vi "Main.vi"() -> ()   [LabVIEW 2017]
doc: "This sample project is built upon the standard state machine template and shows how you could create an application that acquires, analyzes, and presents data. It includes functionality for presenting configuration dialogs, preserving settings between executions, loading and saving data, as well as exporting graph images and text files.\n\nIt is most appropriate for data that is acquired instantly as it does not allow for screen updates mid acquisition nor does it allow for continuous streaming to disk."
uses:
  controls/State.ctl
  controls/Data.ctl
  controls/UI References.ctl
  controls/Graph Data.ctl
  <vilib>/Utility/miscctls.llb/LVAnnotationListTypeDef.ctl
  <vilib>/Utility/miscctls.llb/LVCursorListTypeDef.ctl
  controls/User Specified Data.ctl
  controls/HW Configuration.ctl
  original/controls/Simulated Signal Type.ctl
  controls/Analysis Configuration.ctl
  controls/New Data Behavior.ctl
  <extravilib>/ChannelInstances/Event Messenger-a[.](str)/Instantiate.vi
  <extravilib>/ChannelInstances/Event Messenger-a[.](str)/))Channel.vi
  <extravilib>/ChannelInstances/Event Messenger-str/Instantiate.vi
  <extravilib>/ChannelInstances/Event Messenger-str/))Channel.vi
  subVIs/Settings Dialog.vi
  <extravilib>/ChannelInstances/Event Messenger-str.lvlib
  <extravilib>/ChannelInstances/Event Messenger-a[.](str).lvlib
panel:
  in  "Settings":bool
  in  "Snapshot":bool
  in  "Analyze":bool
  in  "Clear":bool
  in  "Exit":bool
  in  "Acquire":bool
  in  "Export":bool
  in  "Save Data":bool
  in  "Load Data":bool
  out "Graph":waveform(dbl)[](graph)
  out "Status Bar":string
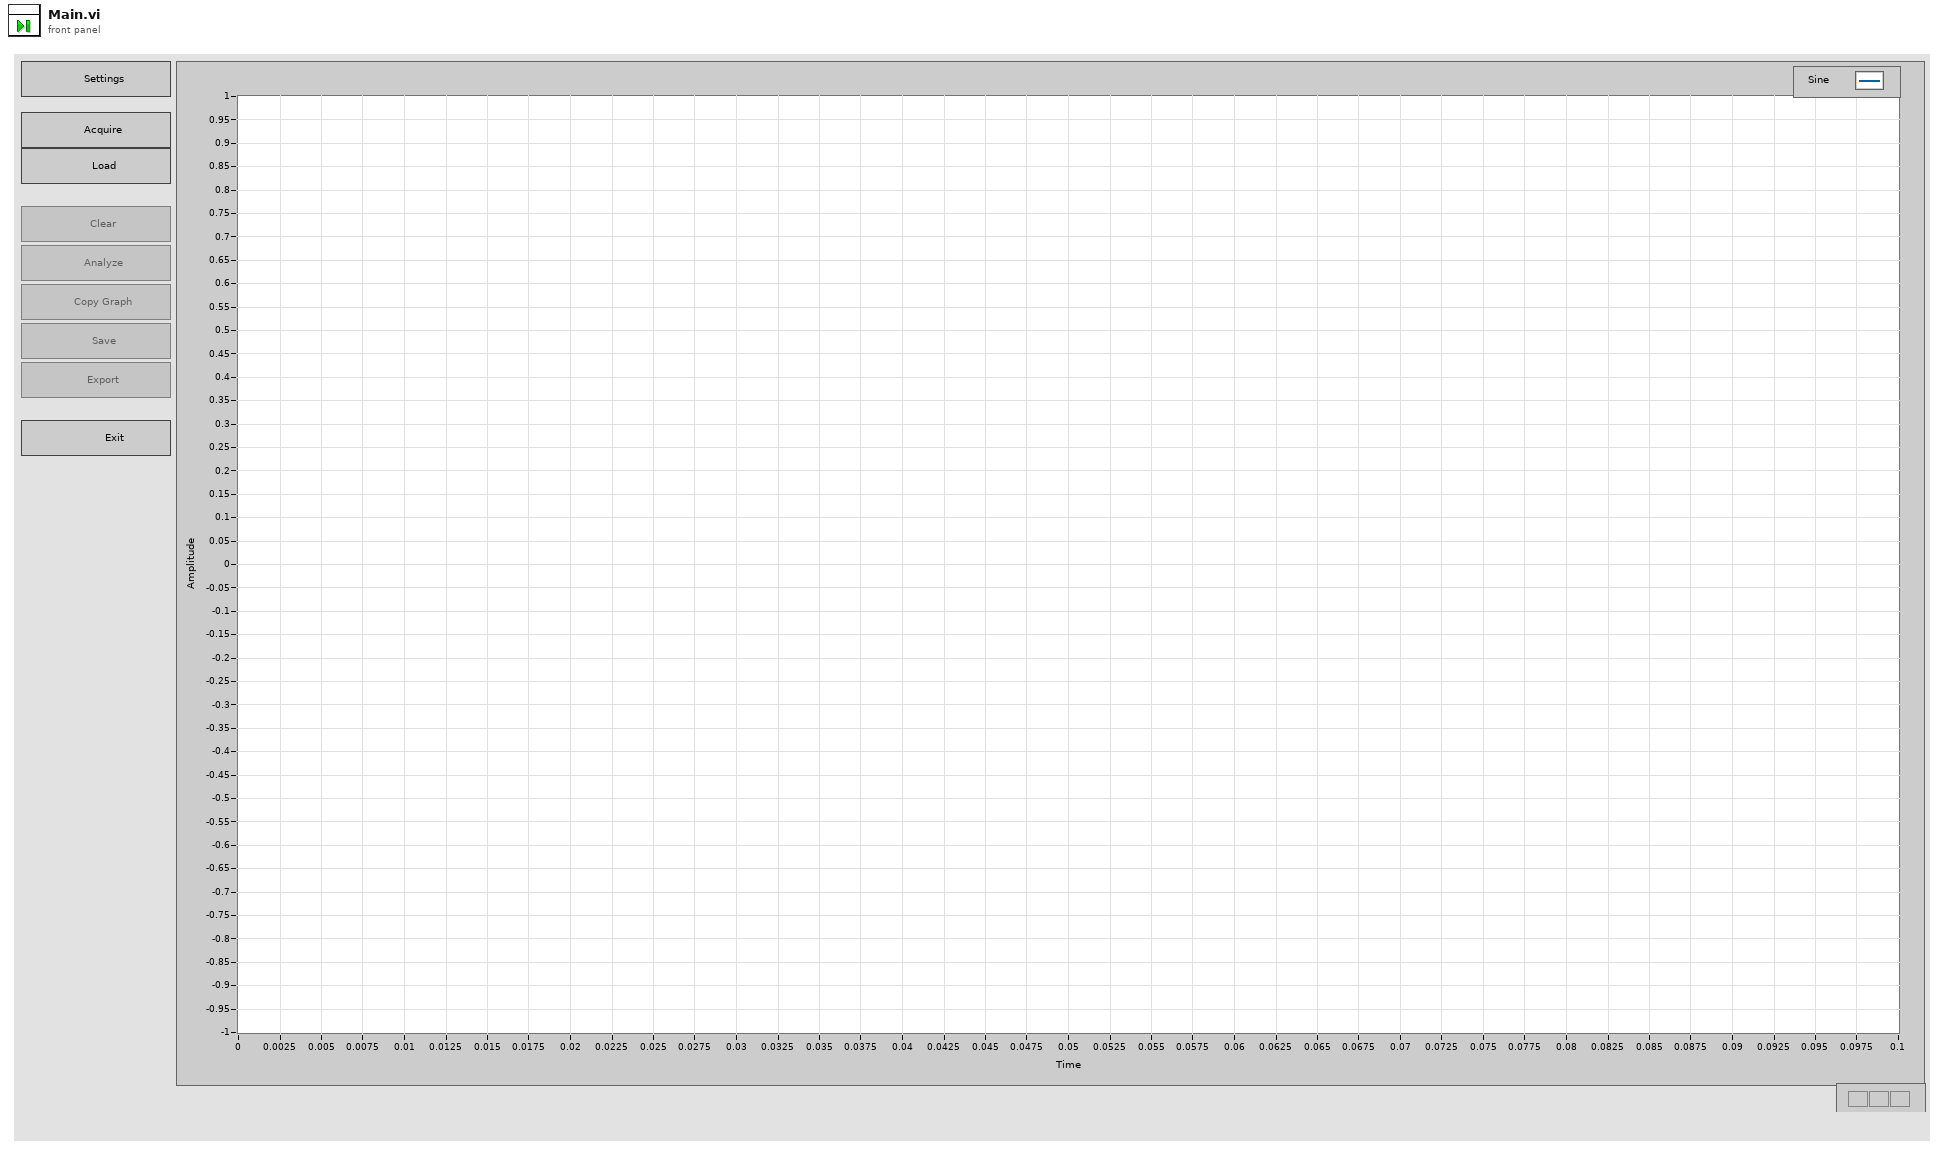
[diagram p1: front panel]
types:
  T1 = typedef "Data.ctl" = cluster{"UI References":T2, "Graph Data":T3, "User Specified":T6}
  T2 = typedef "UI References.ctl" = cluster{"Exit Ref":refnum<vi>, "Save Ref":refnum<vi>, "Open Ref":refnum<vi>, "Export Ref":refnum<vi>, "Acquire Ref":refnum<vi>, "Configure Ref":refnum<vi>, "Graph Ref":refnum<vi>, "Clear Ref":refnum<vi>, "Analyze Ref":refnum<vi>, "Status Ref":refnum<vi>, "Snapshot Ref":refnum<vi>}
  T3 = typedef "Graph Data.ctl" = cluster{"Data":waveform(dbl)[], "Annotation List":T4, "Cursor List":T5, "Analysis Data":waveform(dbl)[]}
  T4 = typedef "LVAnnotationListTypeDef.ctl" = cluster{"Name":string, "Color":u32, "Style":u8, "Point Style":u8, "Name Visible":bool, "Allow Drag":bool, "Annotation Mode":u32, "Plot":i32, "Index":i32, "Position":cluster{"X":dbl, "Y":dbl}, "X Scale":u32, "Y Scale":u32, "Show Arrow":bool, "Lock Name":bool, "Plot Area":i32, "Label Offset":cluster{"X":dbl, "Y":dbl}}[]
  T5 = typedef "LVCursorListTypeDef.ctl" = cluster{"Name":string, "Color":u32, "Style":u8, "Point Style":u8, "Name Visible":bool, "Allow Drag":bool, "Cursor Mode":u32, "Plot":i32, "Index":i32, "Position":cluster{"X":dbl, "Y":dbl}, "X Scale":u32, "Y Scale":u32, "Watch Plots":i32[], "Watch All Plots":bool, "Plot Area":i32, "Label Offset":cluster{"X":dbl, "Y":dbl}}[]
  T6 = typedef "User Specified Data.ctl" = cluster{"Hardware Configuration":T7, "Analysis Configuration":T9, "New Data Behavior":T10, "Signal Configuration":cluster{"I/O Limit":dbl, "Sample Rate":dbl, "Chirp Duration (s)":dbl, "Upper Frequency":dbl, "Lower Frequency":dbl, "Chirp Amplitude":dbl, "Windowing":enum16{"None", "Exponential", "Flat top", "Hamming", "Hanning", "Kaiser-Bessel", "Rectangular"}}}
  T7 = typedef "HW Configuration.ctl" = cluster{"Signal Channel":tag, "Response Channel":tag, "Trigger Channel":tag, "HW Refnum <Replace Me>":string, "Signal Type <Replace Me>":T8}
  T8 = typedef "Simulated Signal Type.ctl" = enum16{"Sine Wave", "Square Wave"}
  T9 = typedef "Analysis Configuration.ctl" = cluster{"Statistics":bool}
  T10 = typedef "New Data Behavior.ctl" = enum16{"Replace", "Overlay", "Append"}
  T11 = typedef "State.ctl" = enum16{"Initialize", "Wait for Event", "Update UI", "Configure", "Acquire", "Load Data", "Save Data", "Clear Data", "Export Data", "Analyze", "Copy Graph", "Exit"}
  T12 = enum16{"Standard", "Buffered", "CRLF", "Immediate"}
  T13 = typedef "Event Messenger-str.lvlib/))Channel.ctl" = refnum<queue>
  T14 = typedef "Event Messenger-a[.](str).lvlib/))Channel.ctl" = refnum<queue>
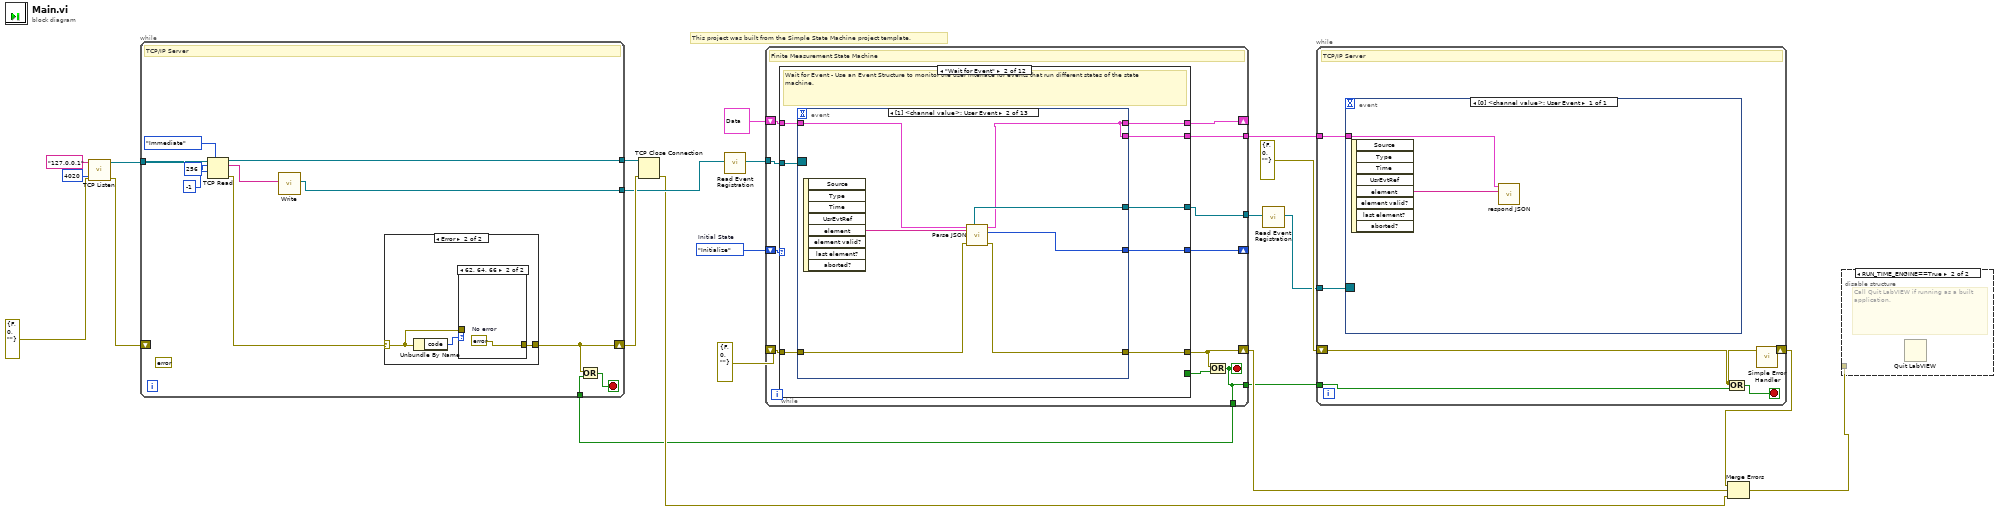
[diagram p0: block diagram]
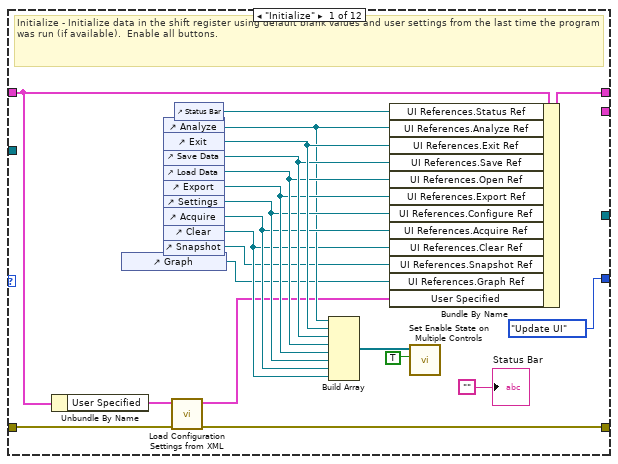
[diagram p5: hidden frame]
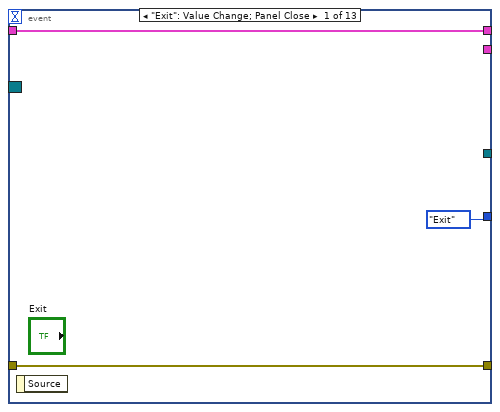
[diagram p6: hidden frame]
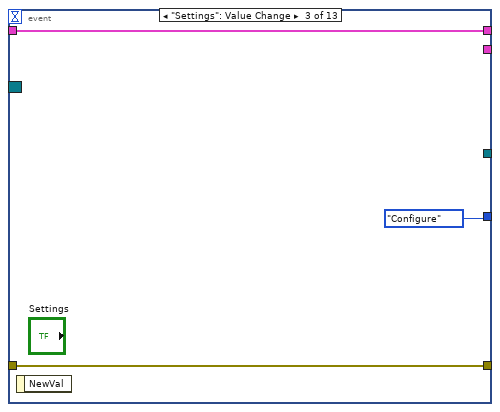
[diagram p7: hidden frame]
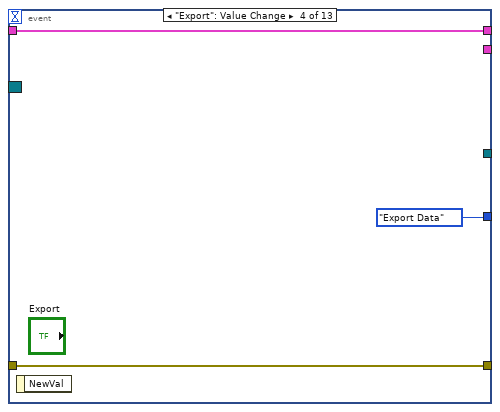
[diagram p8: hidden frame]
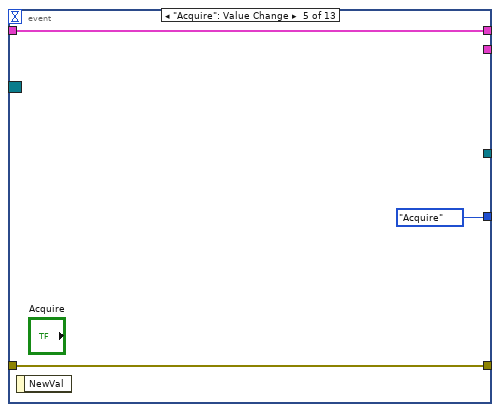
[diagram p9: hidden frame]
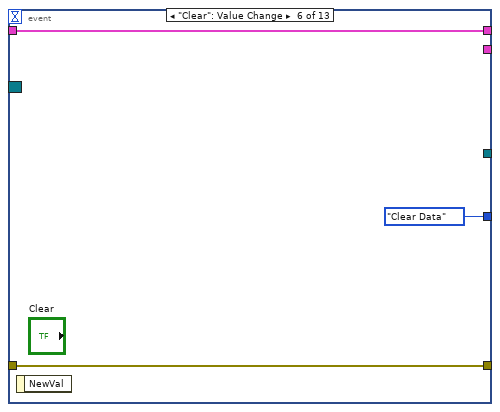
[diagram p10: hidden frame]
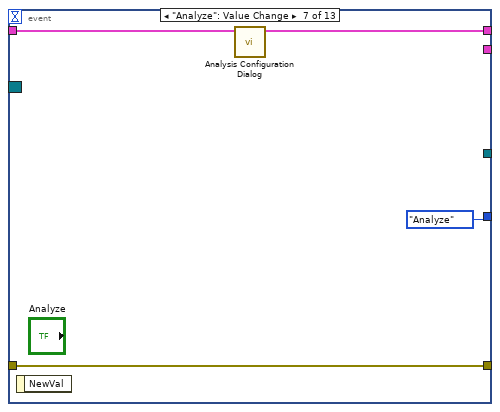
[diagram p11: hidden frame]
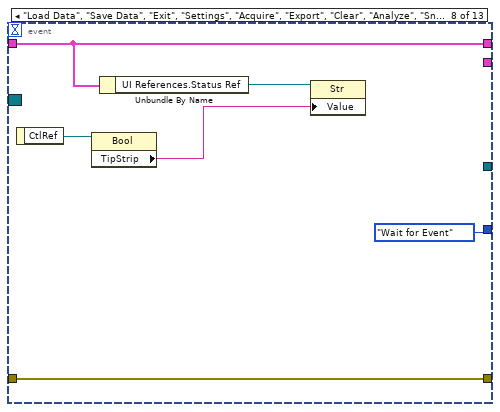
[diagram p12: hidden frame]
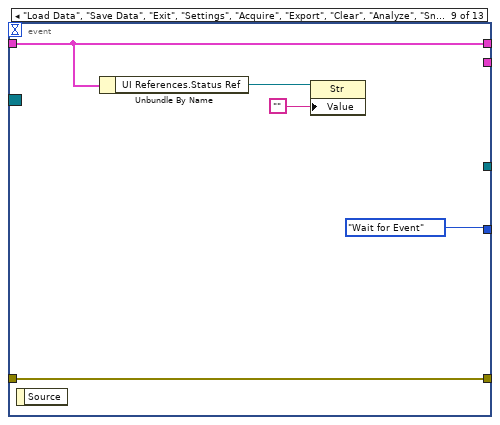
[diagram p13: hidden frame]
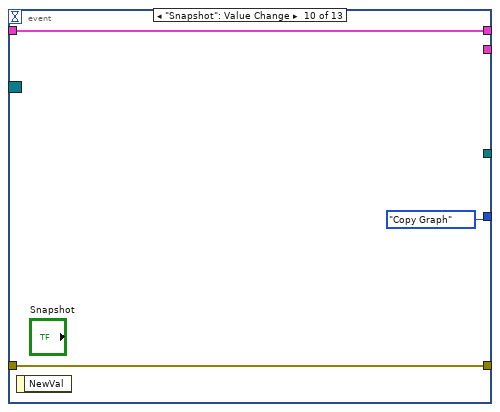
[diagram p14: hidden frame]
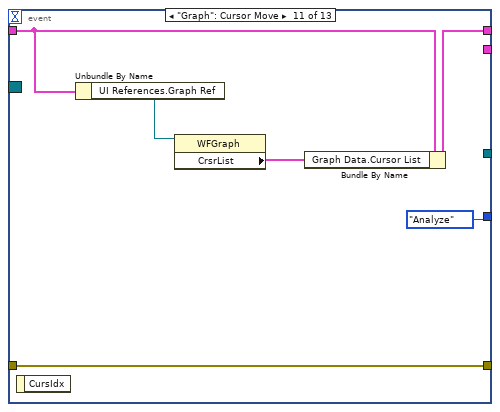
[diagram p15: hidden frame]
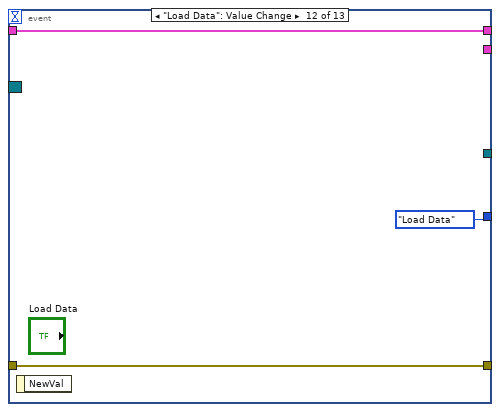
[diagram p16: hidden frame]
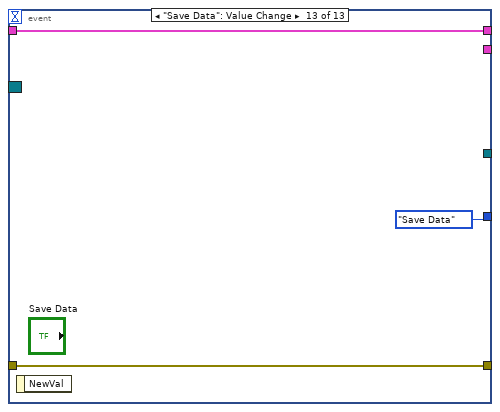
[diagram p17: hidden frame]
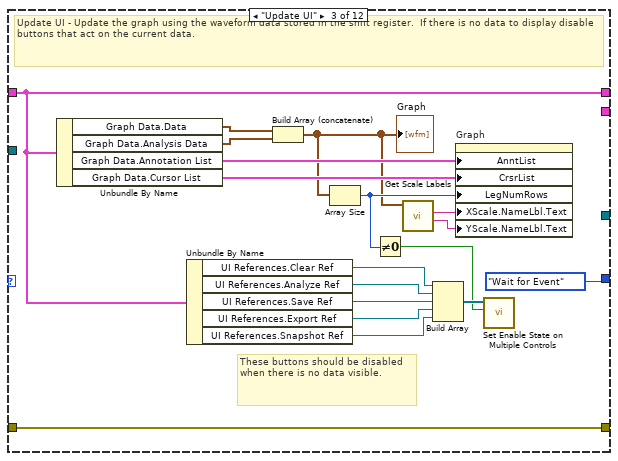
[diagram p18: hidden frame]
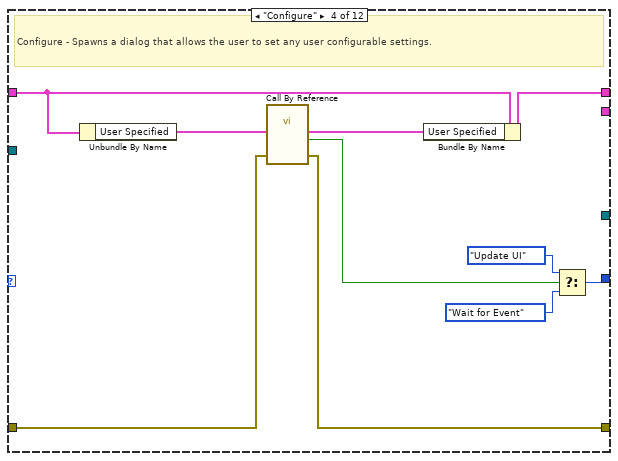
[diagram p19: hidden frame]
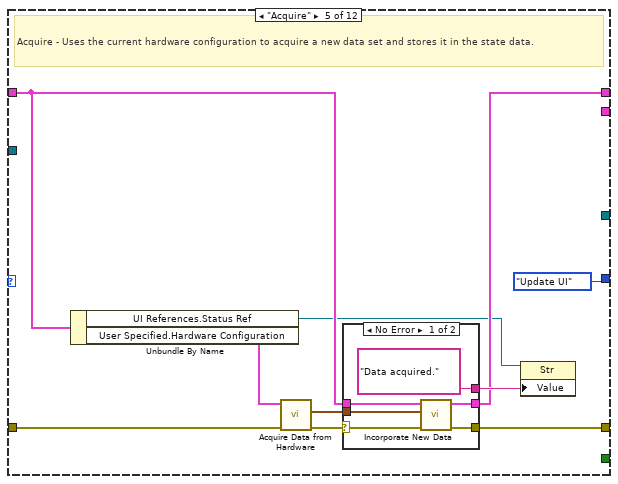
[diagram p20: hidden frame]
diagram:
  (unwired) errorcluster {"status"=FALSE, "code"=0, "source"=""} ("error constant")
  w22 = State."Initialize"  # Initial State
  # "This project was built from the Simple State Machine project template."
  n1 = call <vilib>:"TCP Listen.vi"("error in (no error)"=errorcluster {"status"=FALSE, "code"=0, "source"=""} ("error constant"), "port"=u16 4020 ("remote port or service name"), "service name"="127.0.0.1" ("address")) -> ("error out"=w11:errorcluster, "connection ID"=w18:refnum<k5>)  [unwired: 4 in, 3 out]
  n2 = call <vilib>:"Simple Error Handler.vi"() -> ()  [unwired: 5 in, 5 out]
  n3 = while {
    tunnel: w18 -> [w32]
    tunnel: [w28] -> w17
    tunnel: [w26] -> w15
    shift-right: [w24] -> w16
    shift-left: w11 -> [_]
    tunnel: w1 -> [w23]
    stop <- w33 stop-if-true
    # "TCP/IP Server"
    n4 = TCP Read(connection ID=w32, bytes to read=256, 7:T12."Immediate" ("mode (standard)"), 9:-1 ("timeout ms (25000)")) -> (connection ID out=w28:refnum<k5>, data out=w27:string, error out=w25:errorcluster)  [unwired: 1 in]
    n5 = call <extravilib>:"Write.vi"("element"=w27) -> ("channel"=w26:T13)  [unwired: 9 in, 1 out]
    n6 = case shown="Error" w25 {
      selector: w25 -> [w34 w35]
      tunnel: [w34 w36] -> w24
      frame No Error {
      }
      frame Error {
        n7 = Unbundle By Name(w35) -> ("code"=w37:i32)
        n8 = case shown="62, 64, 66" w37 {
          tunnel: [w38 w39] -> w36
          tunnel: w35 -> [w38 _]
          frame 0, Default {
          }
          frame 62, 64, 66 {
            w39 = errorcluster {"status"=FALSE, "code"=0, "source"=""}  # No error
          }
        }
      }
    }
    n9 = Or(x=w24, y=w23) -> (x .or. y?=w33:bool)
  }
  n10 = TCP Close Connection(connection ID=w17, error in (no error)=w16) -> (error out=w8:errorcluster)  [unwired: 2 out]
  n11 = call <extravilib>:"Read Event Registration.vi"("channel"=w15) -> ("event registration refnum"=w14:refnum<event-registration>)  [unwired: 10 in]
  n12 = while {
    shift-right: [w42] -> _
    shift-left: w22 -> [w50]
    shift-right: [w48] -> _
    shift-left: T1 {"UI References"={"Exit Ref"=refnum, "Save Ref"=refnum, "Open Ref"=refnum, "Export Ref"=refnum, "Acquire Ref"=refnum, "Configure Ref"=refnum, "Graph Ref"=refnum, "Clear Ref"=refnum, "Analyze Ref"=refnum, "Status Ref"=refnum, "Snapshot Ref"=refnum}, "Graph Data"={"Data"=[], "Annotation List"=[], "Cursor List"=[], "Analysis Data"=[]}, "User Specified"={"Hardware Configuration"={"Signal Channel"="", "Response Channel"="", "Trigger Channel"="", "HW Refnum <Replace Me>"="", "Signal Type <Replace Me>"=enum."Sine Wave"}, "Analysis Configuration"={"Statistics"=TRUE}, "New Data Behavior"=enum."Replace", "Signal Configuration"={"I/O Limit"=10.0, "Sample Rate"=1000000.0, "Chirp Duration (s)"=0.01, "Upper Frequency"=0.0, "Lower Frequency"=0.0, "Chirp Amplitude"=0.1, "Windowing"=enum."None"}}} ("Data") -> [w49]
    shift-right: [w45] -> w7
    shift-left: errorcluster {"status"=FALSE, "code"=0, "source"=""} ("error constant") -> [w47]
    tunnel: w14 -> [w44]
    tunnel: [w43] -> w5
    tunnel: [w41] -> w3
    tunnel: [w40] -> w2
    tunnel: [w40] -> w1
    stop <- w40 stop-if-true
    # "Finite Measurement State Machine"
    n13 = case shown="\"Wait for Event\"" w50 {
      tunnel: [_ w79 _ _ _ _ _ _ _ _ _ _] -> w43
      tunnel: [_ _ _ _ _ _ _ _ _ _ _ w241] -> w46
      tunnel: w49 -> [w63 w78 w147 w159 w166 w187 w201 w213 w224 w227 w233 w239]
      tunnel: [w71 w77 w147 w158 w165 w182 w201 w213 w223 w227 w233 w239] -> w48
      tunnel: w47 -> [w61 w76 w149 w157 w168 w186 w203 w216 w225 w228 w232 w236]
      tunnel: [w60 w75 w149 w156 w161 w185 w199 w210 w225 w228 w231 w235] -> w45
      tunnel: w44 -> [_ w74 _ _ _ _ _ _ _ _ _ _]
      tunnel: [State."Update UI" ("Next State") w73 State."Wait for Event" ("(Value Not Used)") w150 State."Update UI" ("Next State") State."Update UI" ("(Value Not Used)") State."Wait for Event" ("(Value Not Used)") State."Wait for Event" ("(Value Not Used)") State."Update UI" ("(Value Not Used)") State."Update UI" ("(Value Not Used)") State."Wait for Event" ("(Value Not Used)") w234] -> w42
      tunnel: [_ w72 _ _ _ _ _ _ _ _ _ _] -> w41
      frame "Initialize" {
        # "Initialize - Initialize data in the shift register using default blank values and user settings from the last time the program was run (if available).  Enable all buttons."
        n14 = Unbundle By Name(w63) -> ("User Specified"=w62:T6)
        n15 = control-ref of="Graph"() -> (w52:refnum<vi>)
        n16 = control-ref of="Analyze"() -> (w59:refnum<vi>)
        n17 = control-ref of="Exit"() -> (w70:refnum<vi>)
        n18 = control-ref of="Save Data"() -> (w69:refnum<vi>)
        n19 = control-ref of="Load Data"() -> (w68:refnum<vi>)
        n20 = control-ref of="Export"() -> (w67:refnum<vi>)
        n21 = control-ref of="Settings"() -> (w66:refnum<vi>)
        n22 = control-ref of="Acquire"() -> (w65:refnum<vi>)
        n23 = control-ref of="Clear"() -> (w57:refnum<vi>)
        n24 = control-ref of="Snapshot"() -> (w53:refnum<vi>)
        n25 = call "Load Configuration Settings from XML.vi"("error in (no error)"=w61, "User Configuration in"=w62) -> ("error out"=w60:errorcluster, "User Configuration out"=w55:T6)  [unwired: 8 in]
        n26 = control-ref of="Status Bar"() -> (w58:refnum<vi>)
        n27 = Build Array(w59, w70, w69, w68, w67, w66, w65, w57) -> (w64:refnum<vi>[])
        n28 = Bundle By Name(cluster=w63, "UI References.Status Ref"=w58, "UI References.Analyze Ref"=w59, "UI References.Exit Ref"=w70, "UI References.Save Ref"=w69, "UI References.Open Ref"=w68, "UI References.Export Ref"=w67, "UI References.Configure Ref"=w66, "UI References.Acquire Ref"=w65, "UI References.Clear Ref"=w57, "UI References.Snapshot Ref"=w53, "UI References.Graph Ref"=w52, "User Specified"=w55) -> (w71:T1)
        n29 = call "Set Enable State on Multiple Controls.vi"("Enable?"=TRUE, "Controls"=w64) -> ()  [unwired: 10 in]
        "Status Bar" <- "" ("Status Bar")
      }
      frame "Wait for Event" {
        # "Wait for Event - Use an Event Structure to monitor the user interface for events that run different states of the state machine."
        n30 = event shown="[1] <channel value>: User Event" {
          selector: w74 -> [_ _ _ _ _ _ _ _ _ _ _ _ _]
          dyn-events: _ -> [_ _ _ _ _ _ _ _ _ _ _ _ _]
          timeout: _ -> [_ _ _ _ _ _ _ _ _ _ _ _ _]
          tunnel: [_ w85 _ _ _ _ _ _ _ _ _ _ _] -> w79
          tunnel: w78 -> [w82 w88 w92 w95 w98 w101 w104 w109 w115 w119 w121 w128 w131]
          tunnel: [w82 w83 w92 w95 w98 w101 w103 w109 w115 w119 w124 w128 w131] -> w77
          tunnel: w76 -> [w81 w87 w91 w94 w97 w100 w105 w111 w116 w118 w125 w127 w130]
          tunnel: [w81 w86 w91 w94 w97 w100 w105 w111 w116 w118 w125 w127 w130] -> w75
          tunnel: [State."Exit" ("Next State") w84 State."Configure" ("Next State") State."Export Data" ("Next State") State."Acquire" ("Next State") State."Clear Data" ("Next State") State."Analyze" ("Next State") State."Wait for Event" ("Next State") State."Wait for Event" ("Next State") State."Copy Graph" ("Next State") State."Analyze" ("Next State") State."Load Data" ("Next State") State."Save Data" ("Next State")] -> w73
          tunnel: [_ w83 _ _ _ _ _ _ _ _ _ _ _] -> w72
          event "Exit": Value Change; Panel Close {
            n31 = event-data() -> ()  [unwired: 1 in, 1 out]
          }
          event User Event {
            n32 = event-data() -> ("element"=w89:string)  [unwired: 1 in, 7 out]
            n33 = call "Parse JSON.vi"("error in (no error)"=w87, "element"=w89, "Data In"=w88) -> ("error in (no error) 2"=w86:errorcluster, "States"=w84:T11, "Data Out"=w83:T1, "Message Channel"=w85:T14)  [unwired: 3 in]
          }
          event "Settings": Value Change {
            n34 = event-data() -> ()  [unwired: 1 in, 1 out]
          }
          event "Export": Value Change {
            n35 = event-data() -> ()  [unwired: 1 in, 1 out]
          }
          event "Acquire": Value Change {
            n36 = event-data() -> ()  [unwired: 1 in, 1 out]
          }
          event "Clear": Value Change {
            n37 = event-data() -> ()  [unwired: 1 in, 1 out]
          }
          event "Analyze": Value Change {
            n38 = event-data() -> ()  [unwired: 1 in, 1 out]
            n39 = call "Analysis Configuration Dialog.vi"("Data in"=w104) -> ("Data out"=w103:T1)  [unwired: 10 in]
          }
          event "Load Data", "Save Data", "Exit", "Settings", "Acquire", "Export", "Clear", "Analyze", "Snapshot": Mouse Enter {
            n40 = event-data() -> ("CtlRef"=w110:refnum<vi>)  [unwired: 1 in]
            n41 = property class="Bool"(reference=w110) -> ("TipStrip"=w107:string)  [unwired: 1 in, 2 out]
            n42 = Unbundle By Name(w109) -> ("UI References.Status Ref"=w108:refnum<vi>)
            n43 = property class="Str"(reference=w108, "Value"=w107) -> ()  [unwired: 1 in, 2 out]
          }
          event "Load Data", "Save Data", "Exit", "Settings", "Acquire", "Export", "Clear", "Analyze", "Snapshot": Mouse Leave {
            n44 = event-data() -> ()  [unwired: 1 in, 1 out]
            n45 = Unbundle By Name(w115) -> ("UI References.Status Ref"=w114:refnum<vi>)
            n46 = property class="Str"(reference=w114, "Value"="") -> ()  [unwired: 1 in, 2 out]
          }
          event "Snapshot": Value Change {
            n47 = event-data() -> ()  [unwired: 1 in, 1 out]
          }
          event "Graph": Cursor Move {
            n48 = event-data() -> ()  [unwired: 1 in, 1 out]
            n49 = Unbundle By Name(w121) -> ("UI References.Graph Ref"=w123:refnum<vi>)
            n50 = property class="WFGraph"(reference=w123) -> ("CrsrList"=w122:T5)  [unwired: 1 in, 2 out]
            n51 = Bundle By Name(cluster=w121, "Graph Data.Cursor List"=w122) -> (w124:T1)
          }
          event "Load Data": Value Change {
            n52 = event-data() -> ()  [unwired: 1 in, 1 out]
          }
          event "Save Data": Value Change {
            n53 = event-data() -> ()  [unwired: 1 in, 1 out]
          }
        }
      }
      frame "Update UI" {
        # "These buttons should be disabled when there is no data visible."
        # "Update UI - Update the graph using the waveform data stored in the shift register.  If there is no data to display disable buttons that act on the current data."
        n54 = Unbundle By Name(w147) -> ("Graph Data.Data"=w143:waveform(dbl)[], "Graph Data.Analysis Data"=w133:waveform(dbl)[], "Graph Data.Annotation List"=w148:T4, "Graph Data.Cursor List"=w144:T5)
        n55 = Unbundle By Name(w147) -> ("UI References.Clear Ref"=w139:refnum<vi>, "UI References.Analyze Ref"=w138:refnum<vi>, "UI References.Save Ref"=w146:refnum<vi>, "UI References.Export Ref"=w136:refnum<vi>, "UI References.Snapshot Ref"=w137:refnum<vi>)
        n56 = Build Array (concatenate)(w143, w133) -> (w141:waveform(dbl)[])
        "Graph" <- w141
        n57 = Array Size(array=w141) -> (size(s)=w142:i32)
        n58 = Not Equal To 0?(x=w142) -> (x != 0?=w140:bool)
        n59 = call "Get Scale Labels.vi"("Array of Waveforms"=w141) -> ("Y Scale Label Text"=w134:string, "X Scale Label Text"=w135:string)  [unwired: 9 in]
        n60 = Build Array(w139, w138, w146, w136, w137) -> (w145:refnum<vi>[])
        n61 = property on="Graph" class="WFGraph (strict)"("AnntList"=w148, "CrsrList"=w144, "LegNumRows"=w142, "XScale.NameLbl.Text"=w135, "YScale.NameLbl.Text"=w134) -> ()  [unwired: 2 in, 2 out]
        n62 = call "Set Enable State on Multiple Controls.vi"("Enable?"=w140, "Controls"=w145) -> ()  [unwired: 10 in]
      }
      frame "Configure" {
        # "Configure - Spawns a dialog that allows the user to set any user configurable settings."
        n63 = Unbundle By Name(w159) -> ("User Specified"=w152:T6)
        n64 = call-by-ref "?"("error in (no error)"=w157, "Configuration in"=w152) -> ("error out"=w156:errorcluster, "UI Refresh Needed?"=w155:bool, "Configuration out"=w151:T6)  [unwired: 9 in, 2 out]
        n65 = Bundle By Name(cluster=w159, "User Specified"=w151) -> (w158:T1)
        n66 = Select(t=State."Update UI" ("Next State if true"), s=w155, f=State."Wait for Event" ("Next State if false")) -> (s? t:f=w150:T11)
      }
      frame "Acquire" {
        # "Acquire - Uses the current hardware configuration to acquire a new data set and stores it in the state data."
        n67 = Unbundle By Name(w166) -> ("UI References.Status Ref"=w162:refnum<vi>, "User Specified.Hardware Configuration"=w169:T7)
        n68 = call "Acquire Data from Hardware.vi"("error in (no error)"=w168, "Hardware Configuration"=w169) -> ("error out"=w163:errorcluster, "Graph Data"=w164:waveform(dbl)[])  [unwired: 8 in]
        n69 = case shown="No Error" w163 {
          selector: w163 -> [w172 w177]
          tunnel: w166 -> [w171 w178]
          tunnel: [w175 w178] -> w165
          tunnel: [w174 _] -> w161
          tunnel: w164 -> [w173 _]
          tunnel: ["Data acquired." ("Data acquired") "Data not acquired." ("Data not acquired")] -> w167
          frame No Error {
            n70 = call "Incorporate New Data.vi"("error in (no error)"=w172, "New Graph Data"=w173, "Data in"=w171) -> ("error out"=w174:errorcluster, "Data out"=w175:T1)  [unwired: 7 in]
          }
          frame Error {
            n71 = call <vilib>:"Simple Error Handler.vi"("error in (no error)"=w177) -> ()  [unwired: 4 in, 5 out]
          }
        }
        n72 = property class="Str"(reference=w162, "Value"=w167) -> ()  [unwired: 1 in, 2 out]
      }
      frame "Load Data" {
        # "Load Data - Loads data from a TDMS file and incorporates it with the existing data according to the user's preference."
        n73 = call "Load Data.vi"("error in (no error)"=w186) -> ("error out"=w184:errorcluster, "New Graph Data"=w181:waveform(dbl)[])  [unwired: 9 in]
        n74 = case shown="No Error" w184 {
          selector: w184 -> [w190 w195]
          tunnel: w187 -> [w189 w196]
          tunnel: [w193 w196] -> w182
          tunnel: [w192 _] -> w185
          tunnel: w181 -> [w191 _]
          tunnel: ["Data loaded." ("Data loaded") "Data not loaded." ("Data not loaded")] -> w183
          frame No Error {
            n75 = call "Incorporate New Data.vi"("error in (no error)"=w190, "New Graph Data"=w191, "Data in"=w189) -> ("error out"=w192:errorcluster, "Data out"=w193:T1)  [unwired: 7 in]
          }
          frame Error {
            n76 = call <vilib>:"Simple Error Handler.vi"("error in (no error)"=w195) -> ()  [unwired: 4 in, 5 out]
          }
        }
        n77 = Unbundle By Name(w182) -> ("UI References.Status Ref"=w180:refnum<vi>)
        n78 = property class="Str"(reference=w180, "Value"=w183) -> ()  [unwired: 1 in, 2 out]
      }
      frame "Save Data" {
        # "Save Data - Saves the existing measurement data to a TDMS file."
        n79 = Unbundle By Name(w201) -> ("UI References.Status Ref"=w200:refnum<vi>, "Graph Data.Data"=w204:waveform(dbl)[])
        n80 = call "Save Data.vi"("error in (no error)"=w203, "Data"=w204) -> ("error out"=w202:errorcluster)  [unwired: 9 in]
        n81 = case shown="No Error" w202 {
          selector: w202 -> [w205 w208]
          tunnel: ["Data saved." ("Data saved") "Data not saved." ("Data not saved")] -> w198
          tunnel: [w205 _] -> w199
          frame No Error {
          }
          frame Error {
            n82 = call <vilib>:"Simple Error Handler.vi"("error in (no error)"=w208) -> ()  [unwired: 4 in, 5 out]
          }
        }
        n83 = property class="Str"(reference=w200, "Value"=w198) -> ()  [unwired: 1 in, 2 out]
      }
      frame "Export Data" {
        # "Export Data - Exports the currently loaded measurement and analysis data to a text file that can be imported into a spreadsheet or other application."
        n84 = Unbundle By Name(w213) -> ("UI References.Status Ref"=w211:refnum<vi>, "Graph Data"=w212:T3)
        n85 = call "Export Data.vi"("error in (no error)"=w216, "Graph Data"=w212) -> ("error out"=w214:errorcluster)  [unwired: 9 in]
        n86 = case shown="No Error" w214 {
          selector: w214 -> [w217 w220]
          tunnel: ["Data exported." ("Data exported") "Data not exported." ("Data not exported")] -> w215
          tunnel: [w217 _] -> w210
          frame No Error {
          }
          frame Error {
            n87 = call <vilib>:"Simple Error Handler.vi"("error in (no error)"=w220) -> ()  [unwired: 4 in, 5 out]
          }
        }
        n88 = property class="Str"(reference=w211, "Value"=w215) -> ()  [unwired: 1 in, 2 out]
      }
      frame "Clear Data" {
        # "Clear Data - Clears the data currently in the graph."
        n89 = Bundle By Name(cluster=w224, "Graph Data"=T3 {"Data"=[], "Annotation List"=[], "Cursor List"=[], "Analysis Data"=[]} ("Graph")) -> (w223:T1)
      }
      frame "Analyze" {
        # "#CodeRecommended - Add your own signal analysis here."
        # "Analyze - Analyzes the measurement data."
        n90 = Unbundle By Name(w227) -> ("Graph Data"=w229:T3)
        n91 = call "Statistical Analysis.vi"("Graph Data In"=w229) -> ()  [unwired: 9 in, 2 out]
      }
      frame "Copy Graph" {
        # "Copy Graph - Places an image of the graph on the clipboard for pasting into reports or emails."
        n92 = call "Copy Graph to Clipboard.vi"("error in (no error)"=w232, "Graph Data"=w233) -> ("error out"=w231:errorcluster)  [unwired: 9 in]
      }
      frame "Exit" {
        w241 = TRUE  # Stop Loop?
        w234 = State."Exit"  # (Value Not Used)
        # "Exit - Saves the user's settings to an XML file and stops execution."
        n93 = Unbundle By Name(w239) -> ("UI References.Status Ref"=w237:refnum<vi>, "User Specified"=w240:T6)
        n94 = call "Save Configuration Settings to XML.vi"("error in (no error)"=w236, "User Configuration"=w240) -> ("error out"=w235:errorcluster)  [unwired: 9 in]
        n95 = property class="Str"(reference=w237, "Value"="Application exit." ("Stopped")) -> ()  [unwired: 1 in, 2 out]
      }
    }
    n96 = Or(x=w45, y=w46) -> (x .or. y?=w40:bool)
  }
  n97 = call <extravilib>:"Read Event Registration.vi"("channel"=w5) -> ("event registration refnum"=w4:refnum<event-registration>)  [unwired: 10 in]
  n98 = while {
    shift-right: [w246] -> w6
    shift-left: errorcluster {"status"=FALSE, "code"=0, "source"=""} ("error constant") -> [w246]
    tunnel: w4 -> [w244]
    tunnel: w3 -> [w243]
    tunnel: w2 -> [w242]
    stop <- w245 stop-if-true
    # "TCP/IP Server"
    n99 = event shown="[0] <channel value>: User Event" {
      selector: w244 -> [_]
      dyn-events: _ -> [_]
      timeout: _ -> [_]
      tunnel: w243 -> [w247]
      event User Event {
        n100 = event-data() -> ("element"=w248:string[])  [unwired: 1 in, 7 out]
        n101 = call "respond JSON.vi"("Array"=w248, "Data In"=w247) -> ()  [unwired: 9 in, 1 out]
      }
    }
    n102 = Or(x=w246, y=w242) -> (x .or. y?=w245:bool)
  }
  n103 = Merge Errors(w6, w7, w8) -> (w9:errorcluster)
  n104 = disable-structure shown="RUN_TIME_ENGINE==True" {
    disable-tunnel: w9 -> [_ _]
    frame condition #0 (active) {
    }
    frame condition #1 {
      # "Call Quit LabVIEW if running as a built application."
      n105 = Quit LabVIEW() -> ()  [unwired: 1 in]
    }
  }
